vi "calc.vi"() -> ()   [LabVIEW 2025]
panel:
  in  "stop":bool
  in  "b":dbl
  in  "a":dbl
  out "o/p":dbl
  in  "Boolean":bool
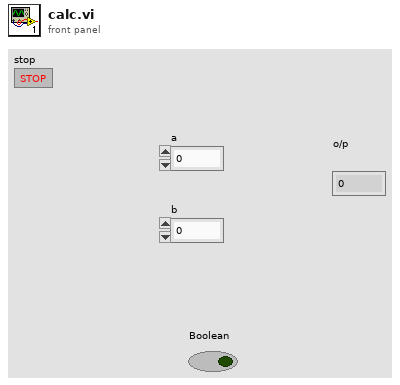
[diagram p1: front panel]
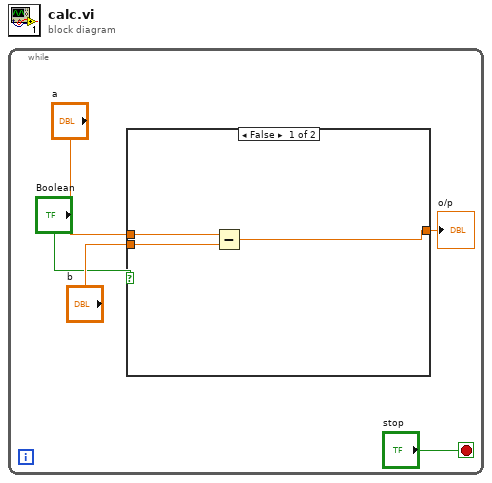
[diagram p0: block diagram]
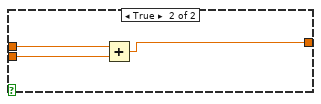
[diagram p2: hidden frame]
diagram:
  n1 = while {
    stop <- "stop" stop-if-true
    n2 = case shown="False" "Boolean" {
      tunnel: "a" -> [w8 w11]
      tunnel: "b" -> [w7 w10]
      tunnel: [w6 w9] -> w3
      frame False {
        n3 = Subtract(x=w8, y=w7) -> (x-y=w6:dbl)
      }
      frame True {
        n4 = Add(x=w11, y=w10) -> (x+y=w9:dbl)
      }
    }
    "o/p" <- w3
  }
